vi "Check if Nest Alias.vi"(9 "Msg Q DVR Alias":string, 10 "Self Actor":refnum<class "Actor.lvclass">) -> (0 "error out":errorcluster, 2 "Used Alias?":bool)   [LabVIEW 2021, in "LVCAM.lvlib" / "Self Actor.lvclass"]
uses:
  Self Actor.lvclass
  Actor/Actor.lvclass
  Self Actor.lvclass/Self Actor.ctl
  LVCAM.lvlib
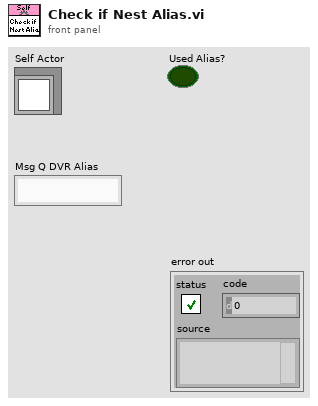
[diagram p1: front panel]
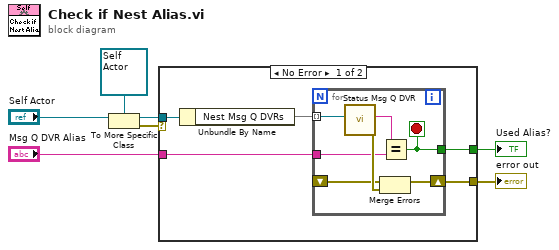
[diagram p0: block diagram]
diagram:
  n1 = To More Specific Class(target class=refnum<class "Self Actor.lvclass"> refnum ("LVCAM.lvlib:Self Actor.lvclass"), reference="Self Actor") -> (specific class reference=w2:refnum<class "Self Actor.lvclass">, error out=w1:errorcluster)  [unwired: 1 in]
  n2 = case shown="No Error" w1 {
    selector: w1 -> [_ w20]
    tunnel: [w11 w20] -> w7
    tunnel: "Msg Q DVR Alias" -> [w10 _]
    tunnel: [w9 _] -> w5
    tunnel: w2 -> [w8 _]
    frame No Error {
      n3 = Unbundle By Name(w8) -> ("Nest Msg Q DVRs"=w12:set{refnum<data-value>})
      n4 = for {
        tunnel: w12 -> [w19] mode=indexing
        shift-right: [w17] -> w11
        shift-left: _ -> [w16]
        tunnel: w10 -> [w14]
        tunnel: [w13] -> w9
        stop <- w13 stop-if-true
        n5 = call "Status Msg Q DVR.vi"("Msg Q DVR"=w19) -> ("error out"=w18:errorcluster, "Msg Q DVR Alias"=w15:string)  [unwired: 9 in]
        n6 = Merge Errors(w16, w18) -> (w17:errorcluster)
        n7 = Equal?(x=w15, y=w14) -> (x = y?=w13:bool)
      }
    }
    frame Error {
    }
  }
  "error out" <- w7
  "Used Alias?" <- w5
